vi "PD Int.vi"() -> ()   [LabVIEW 2018]
uses:
  <vilib>/Analysis/NI_AALPro.lvlib
panel:
  in  "PD Offset":dbl
  out "PD Signal":dynamicdata(graph)
  out "Laser Frequency":dynamicdata(graph)
  in  "number of samples":i32=5000
  in  "rate":dbl=1000.0
  in  "Filename":path=path "C:/Users/physics-svc-fulda/Desktop/LabVIEW Data/PD Int.lvm"
  out "Saving Data":bool
  in  "Enable":bool=TRUE
  out "PD Int":dynamicdata(graph)
  in  "timeout (s)":dbl=10.0 format="%0.2f"
  # "Area Under PD Signal"
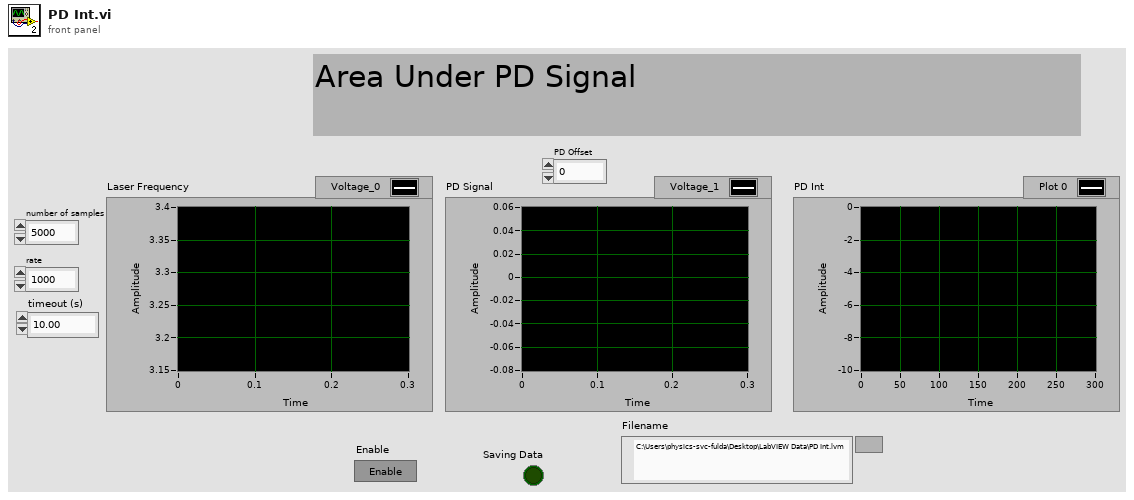
[diagram p1: front panel]
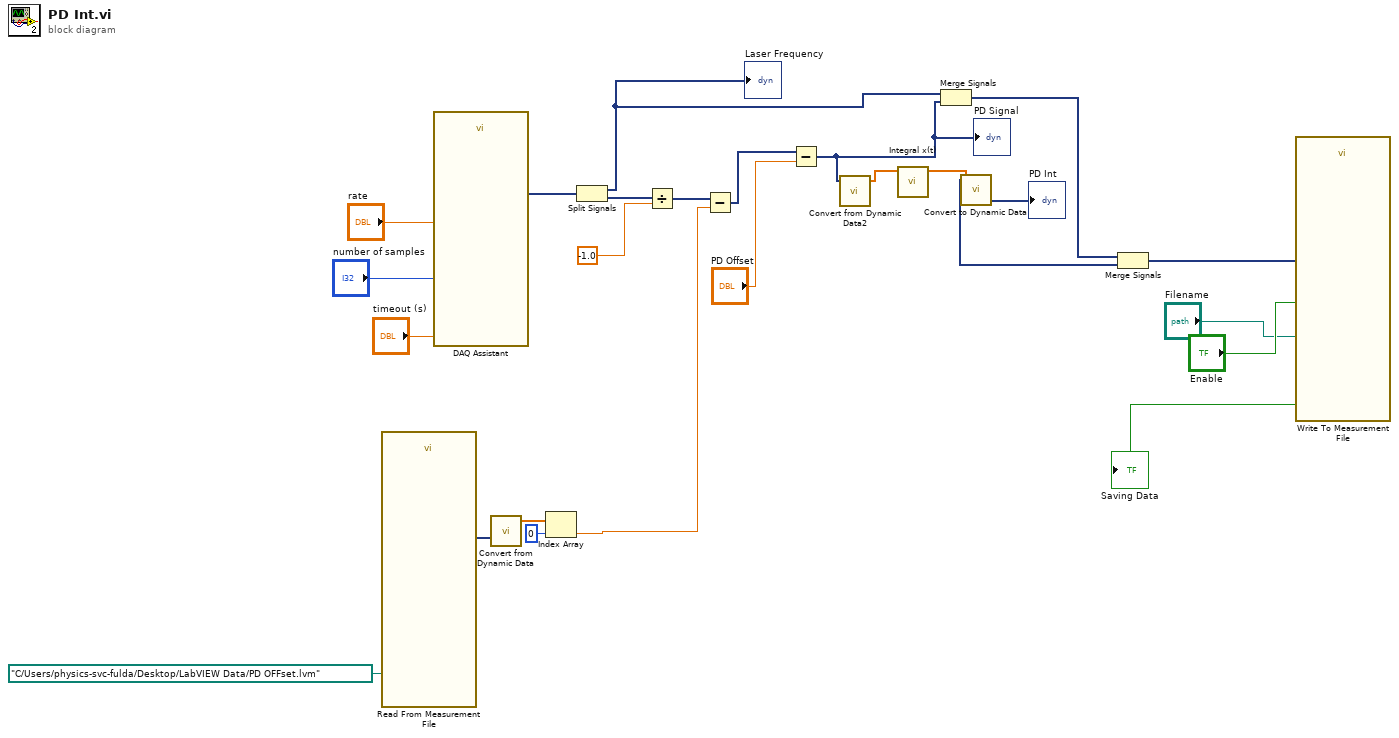
[diagram p0: block diagram]
diagram:
  n1 = call "Read From Measurement File"("Filename"=path "C:/Users/physics-svc-fulda/Desktop/LabVIEW Data/PD OFFset.lvm") -> ("Signals"=w21:dynamicdata)  [unwired: 5 in, 5 out]
  n2 = call "DAQ Assistant"("rate"="rate", "number of samples"="number of samples", "timeout (s)"="timeout (s)") -> ("data"=w23:dynamicdata)  [unwired: 14 in, 2 out]
  n3 = call "Convert from Dynamic Data"("Dynamic Data Type"=w21) -> ("Array"=w22:dbl[])  [unwired: 3 in]
  n4 = Index Array(array=w22, index=0) -> (element=w19:dbl)
  n5 = Split Signals(w23) -> (w7:dynamicdata, w6:dynamicdata)  [unwired: 2 in]
  "Laser Frequency" <- w7
  n6 = Divide(x=w6, y=-1.0) -> (x/y=w5:dynamicdata)
  n7 = Subtract(x=w5, y=w19) -> (x-y=w4:dynamicdata)
  n8 = Subtract(x=w4, y="PD Offset") -> (x-y=w1:dynamicdata)
  "PD Signal" <- w1
  n9 = call "Convert from Dynamic Data2"("Dynamic Data Type"=w1) -> ("Array"=w18:dbl[])  [unwired: 3 in]
  n10 = call <vilib>:"Integral x(t).vi"("X"=w18) -> ("Integral X"=w17:dbl[])  [unwired: 9 in, 1 out]
  n11 = Merge Signals(w7, w1) -> (w13:dynamicdata)
  n12 = call "Convert to Dynamic Data"("Array"=w17) -> ("Dynamic Data Type"=w12:dynamicdata)  [unwired: 3 in]
  "PD Int" <- w12
  n13 = Merge Signals(w13, w12) -> (w16:dynamicdata)
  n14 = call "Write To Measurement File"("Signals"=w16, "Enable"="Enable", "Filename"="Filename") -> ("Saving Data"=→"Saving Data":bool)  [unwired: 14 in, 2 out]
